vi "LIST.vi"(8 "error in (no error)":errorcluster, 10 "Remote File":string, 11 "FTP in":refnum<class "FTP.lvclass">) -> (0 "error out":errorcluster, 2 "Dir-File Info Array":T1[](array[typedef]), 3 "FTP out":refnum<class "FTP.lvclass">)   [LabVIEW 2013, in "FTP.lvlib" / "FTP.lvclass"]
uses:
  FTP.lvclass
  controls/Dir-File Type.ctl
  controls/Dir-File Info.ctl
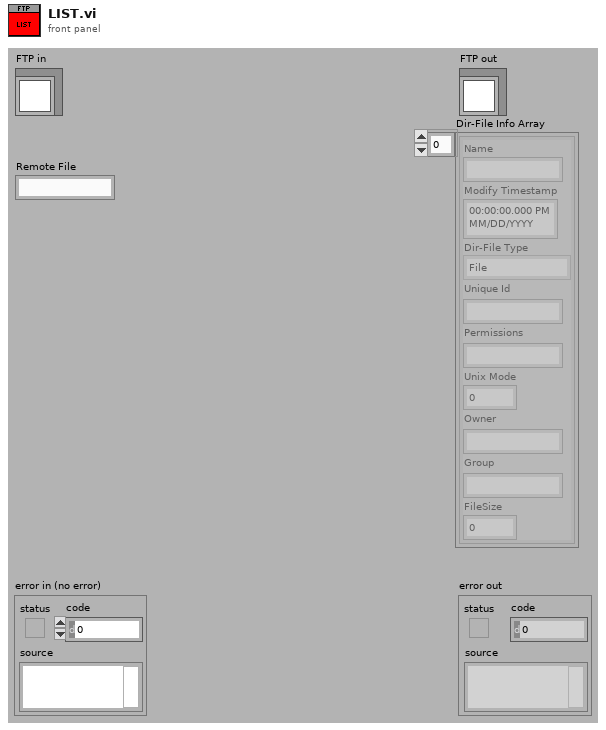
[diagram p1: front panel]
types:
  T1 = typedef "FTP.lvlib/FTP.lvclass/Dir-File Info.ctl" = cluster{"Name":string, "Modify Timestamp":timestamp, "Dir-File Type":T2, "Unique Id":string, "Permissions":string, "Unix Mode":u16, "Owner":string, "Group":string, "FileSize":i64}
  T2 = typedef "FTP.lvlib/FTP.lvclass/Dir-File Type.ctl" = enum16{"File", "Listed Directory", "Parent Directory", "Directory", "Unknown"}
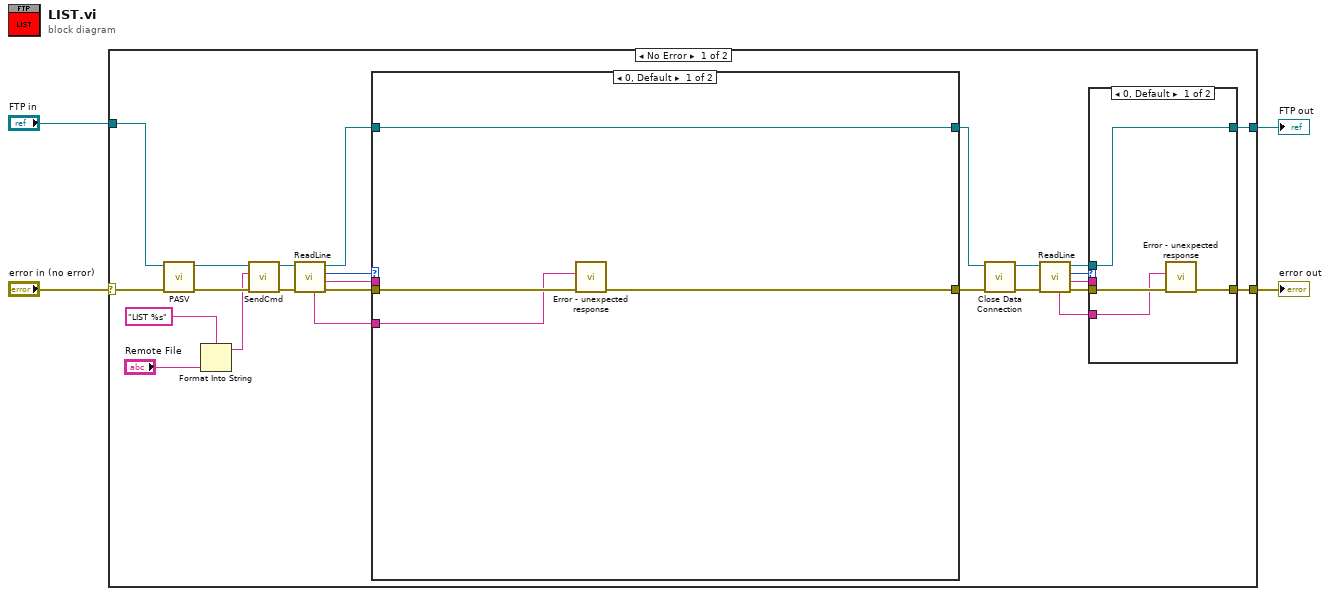
[diagram p0: block diagram]
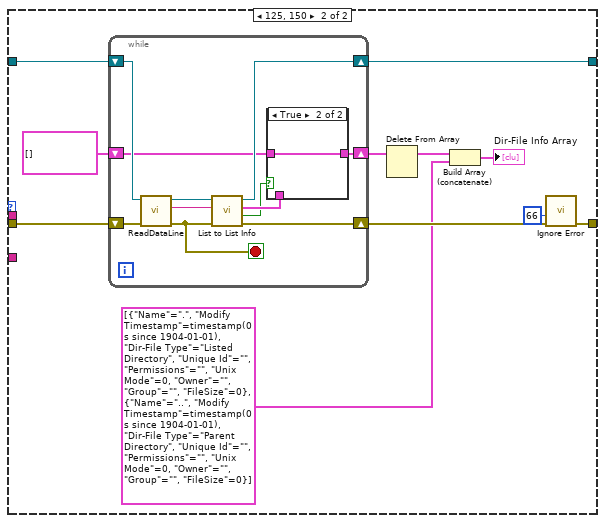
[diagram p3: hidden frame]
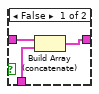
[diagram p4: hidden frame]
diagram:
  n1 = case shown="No Error" "error in (no error)" {
    selector: "error in (no error)" -> [w27 w67]
    tunnel: [w10 w67] -> w3
    tunnel: [w11 w66] -> w1
    tunnel: "FTP in" -> [w26 w66]
    frame No Error {
      n2 = call "PASV.vi"("error in (no error)"=w27, "FTP in"=w26) -> ("error out"=w24:errorcluster, "FTP out"=w25:refnum<class "FTP.lvclass">)  [unwired: 8 in]
      n3 = Format Into String(format string="LIST %s" ("cmd"), "Remote File") -> (resulting string=w7:string)  [unwired: 2 in, 1 out]
      n4 = call "SendCmd.vi"("error in (no error)"=w24, "cmd"=w7, "FTP in"=w25) -> ("error out"=w28:errorcluster, "FTP out"=w29:refnum<class "FTP.lvclass">)  [unwired: 7 in]
      n5 = call "ReadLine.vi"("error in (no error)"=w28, "FTP in"=w29) -> ("error out"=w23:errorcluster, "Line"=w21:string, "code"=w22:i32, "FTP out"=w20:refnum<class "FTP.lvclass">, "Full Line"=w5:string)  [unwired: 5 in]
      n6 = case shown="0, Default" w22 {
        tunnel: w23 -> [w38 w50]
        tunnel: w20 -> [w39 w49]
        tunnel: [w36 w46] -> w13
        tunnel: [w39 w48] -> w12
        tunnel: w21 -> [_ _]
        tunnel: w5 -> [w37 _]
        frame 0, Default {
          n7 = call "Error - unexpected response.vi"("error in (no error)"=w38, "Full Response"=w37) -> ("error out"=w36:errorcluster)  [unwired: 9 in]
        }
        frame 125, 150 {
          n8 = while {
            shift-right: [w58] -> w47
            shift-left: w50 -> [w61]
            shift-right: [w55] -> w48
            shift-left: w49 -> [w60]
            shift-right: [w54] -> w44
            shift-left: T1[] [] -> [w52]
            stop <- w59 stop-if-true
            n9 = call "ReadDataLine.vi"("error in (no error)"=w61, "FTP in"=w60) -> ("error out"=w59:errorcluster, "Data"=w56:string, "FTP out"=w57:refnum<class "FTP.lvclass">)  [unwired: 7 in]
            n10 = call "List to List Info.vi"("error in (no error)"=w59, "List String"=w56, "FTP in"=w57) -> ("error out"=w58:errorcluster, "invalid data"=w51:bool, "Dir-File Info"=w53:T1, "FTP out"=w55:refnum<class "FTP.lvclass">)  [unwired: 5 in]
            n11 = case shown="True" w51 {
              tunnel: [w64 w65] -> w54
              tunnel: w53 -> [w63 _]
              tunnel: w52 -> [w62 w65]
              frame False {
                n12 = Build Array (concatenate)(w62, w63) -> (w64:T1[])
              }
              frame True {
              }
            }
          }
          n13 = Delete From Array(array=w44) -> (array with subset deleted=w43:T1[])  [unwired: 2 in, 1 out]
          n14 = Build Array (concatenate)(w43, T1[] [{"Name"=".", "Modify Timestamp"=timestamp(0 s since 1904-01-01), "Dir-File Type"=enum."Listed Directory", "Unique Id"="", "Permissions"="", "Unix Mode"=0, "Owner"="", "Group"="", "FileSize"=0}, {"Name"="..", "Modify Timestamp"=timestamp(0 s since 1904-01-01), "Dir-File Type"=enum."Parent Directory", "Unique Id"="", "Permissions"="", "Unix Mode"=0, "Owner"="", "Group"="", "FileSize"=0}] ("Dir-File Info Array")) -> (→"Dir-File Info Array":T1[])
          n15 = call "Ignore Error.vi"("error in"=w47, "code"=66) -> ("error out"=w46:errorcluster)  [unwired: 9 in]
        }
      }
      n16 = call "Close Data Connection.vi"("error in (no error)"=w13, "FTP in"=w12) -> ("error out"=w19:errorcluster, "FTP out"=w18:refnum<class "FTP.lvclass">)  [unwired: 8 in]
      n17 = call "ReadLine.vi"("error in (no error)"=w19, "FTP in"=w18) -> ("error out"=w17:errorcluster, "Line"=w14:string, "code"=w16:i32, "FTP out"=w15:refnum<class "FTP.lvclass">, "Full Line"=w6:string)  [unwired: 5 in]
      n18 = case shown="0, Default" w16 {
        tunnel: w17 -> [w32 w34]
        tunnel: [w30 w34] -> w10
        tunnel: w15 -> [w33 w35]
        tunnel: [w33 w35] -> w11
        tunnel: w14 -> [_ _]
        tunnel: w6 -> [w31 _]
        frame 0, Default {
          n19 = call "Error - unexpected response.vi"("error in (no error)"=w32, "Full Response"=w31) -> ("error out"=w30:errorcluster)  [unwired: 9 in]
        }
        frame 226 {
        }
      }
    }
    frame Error {
    }
  }
  "error out" <- w3
  "FTP out" <- w1
